vi "Set Enable State on Multiple Controls.vi"(10 "Activé ?":bool, 11 "Commandes":refnum<vi>[](array[refnum])) -> ()   [LabVIEW 2020]
doc: "Définit toutes les commandes du tableau en entrée à la valeur \"État Activé\"."
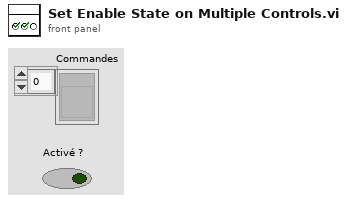
[diagram p1: front panel]
types:
  T1 = enum8{"Enabled", "Disabled", "Disabled and Grayed Out"}
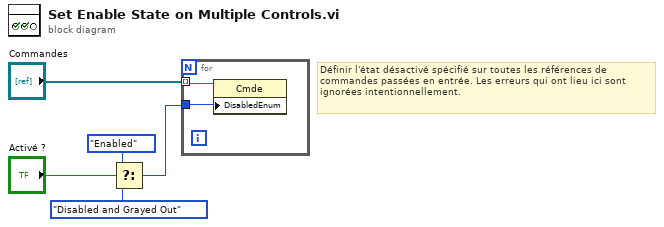
[diagram p0: block diagram]
diagram:
  # "Définir l'état désactivé spécifié sur toutes les références de commandes passées en entrée. Les erreurs qui ont lieu ici sont ignorées intentionnellement."
  n1 = Select(t=T1."Enabled" ("Disabled"), s="Activé ?", f=T1."Disabled and Grayed Out" ("Disabled")) -> (s? t:f=w3:T1)
  n2 = for {
    tunnel: "Commandes" -> [w7] mode=indexing
    tunnel: w3 -> [w6]
    n3 = property class="Cmde"(reference=w7, "DisabledEnum"=w6) -> ()  [unwired: 1 in, 2 out]
  }
